vi "WriteChannels_SingleValue.vi"(4 "Value":bool, 5 "Channels":i32[](array[numeric]), 6 "error in":errorcluster) -> (0 "error out":errorcluster)   [LabVIEW 2014]
doc: "Write value to the specified channels. All channels must be configured as an output before calling this VI."
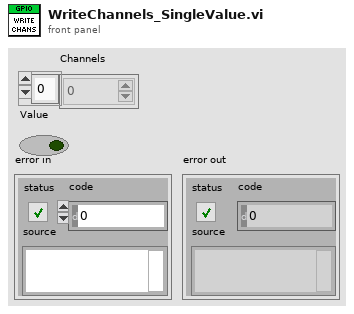
[diagram p1: front panel]
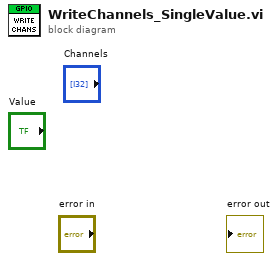
[diagram p0: block diagram]
diagram:
